vi "extract_exe_specific.vi"(8 "error in (no error)":errorcluster, 9 "files_to_extract (relative) []":path[](array[path]), 10 "target_path in":path, 11 "archive_path (file_dialog)":path) -> (0 "error out":errorcluster, 2 "target_path out":path, 3 "archive_path out":path)   [LabVIEW 2015, in "lv-bin-7zip.lvlib" / "v1.lvlib"]
uses:
  v1.lvlib
  lv-bin-7zip.lvlib
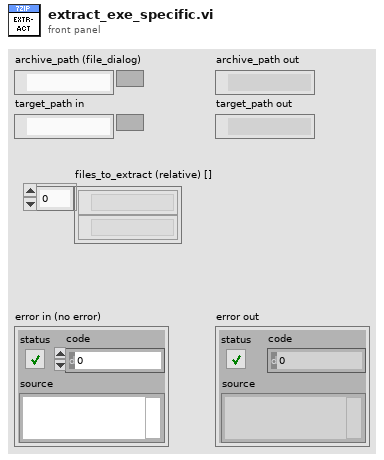
[diagram p1: front panel]
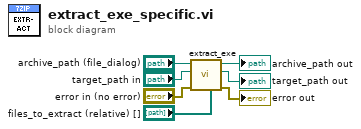
[diagram p0: block diagram]
diagram:
  n1 = call "extract_exe.vi"("files_to_extract (relative) []"="files_to_extract (relative) []", "error in (no error)"="error in (no error)", "target_path in"="target_path in", "archive_path (file_dialog)"="archive_path (file_dialog)") -> ("error out"=→"error out":errorcluster, "target_path out"=→"target_path out":path, "archive_path out"=→"archive_path out":path)  [unwired: 4 in, 1 out]
